vi "Data Cloud Service.vi"(7 "Data Cloud Service Url":string="http://127.0.0.1:8001/DataWS", 8 "Error In":errorcluster, 10 "Data (EU)":dbl[](array[numeric]) format="%.2g") -> (0 "Error Out":errorcluster)   [LabVIEW 2019]
uses:
  <vilib>/httpClient/LabVIEWHTTPClient.lvlib
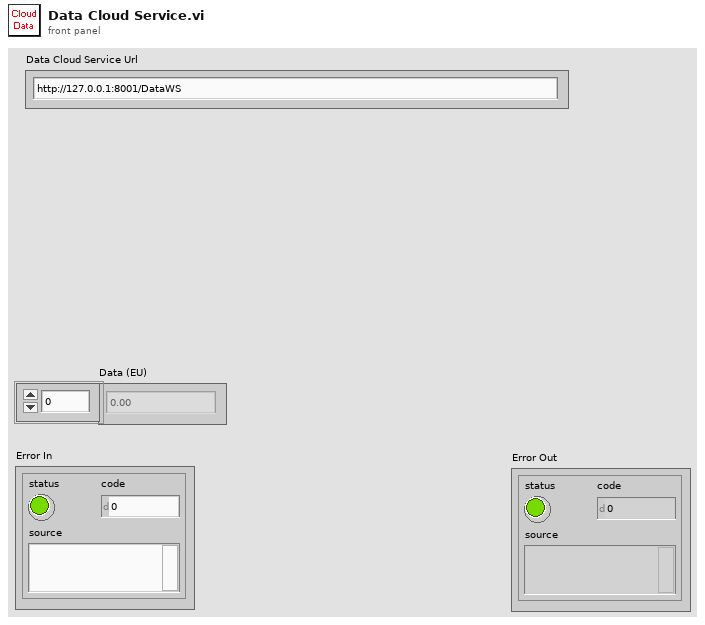
[diagram p1: front panel]
types:
  T1 = typedef "LabVIEWHTTPClient.lvlib/ClientHandle.ctl" = refnum<k1>
  T2 = cluster{"TagId":string, "TagName":string, "TagType":string, "PhysicalChannel":tag, "Vmin":dbl, "Vmax":dbl, "Unit":string, "EUmin":dbl, "EUmax":dbl}[]
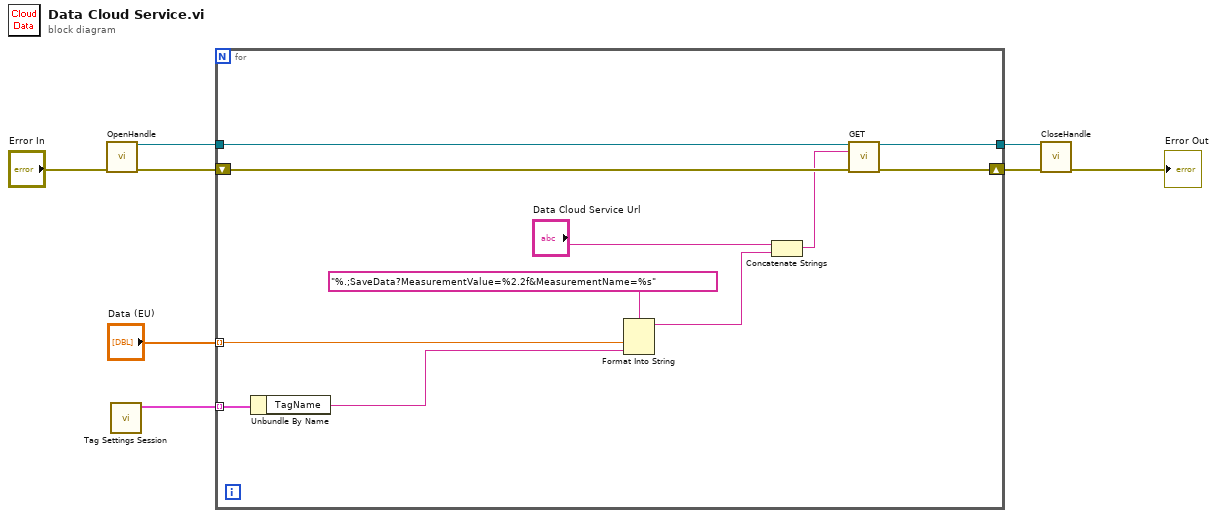
[diagram p0: block diagram]
diagram:
  n1 = call <vilib>:"OpenHandle.vi"("error in (no error)"="Error In") -> ("client handle out"=w7:T1, "error out"=w8:errorcluster)  [unwired: 13 in]
  n2 = call "Tag Settings Session.vi"() -> ("Tag Settings"=w1:T2)  [unwired: 10 in, 1 out]
  n3 = for {
    shift-right: [w16] -> w3
    shift-left: w8 -> [w17]
    tunnel: w7 -> [w19]
    tunnel: "Data (EU)" -> [w18] mode=indexing
    tunnel: w1 -> [w10] mode=indexing
    tunnel: [w15] -> w4
    n4 = Unbundle By Name(w10) -> ("TagName"=w9:string)
    n5 = Format Into String(format string="%.;SaveData?MeasurementValue=%2.2f&MeasurementName=%s" ("url"), w18, w9) -> (resulting string=w11:string)  [unwired: 2 in, 1 out]
    n6 = Concatenate Strings("Data Cloud Service Url", w11) -> (w13:string)
    n7 = call <vilib>:"GET.vi"("client handle"=w19, "url"=w13, "error in (no error)"=w17) -> ("client handle out"=w15:T1, "error out"=w16:errorcluster)  [unwired: 9 in, 2 out]
  }
  n8 = call <vilib>:"CloseHandle.vi"("client handle"=w4, "error in (no error)"=w3) -> ("error out"=→"Error Out":errorcluster)  [unwired: 13 in]
